vi "Page_Advanced_Initialize.vi"(6 "ctl references":T1, 8 "error in (no error)":errorcluster, 11 "AB_Application in":refnum<class "AB_Application.lvclass">) -> (0 "error out":errorcluster, 3 "AB_Application out":refnum<class "AB_Application.lvclass">)   [LabVIEW 2020, in "AB_Application.lvclass"]
uses:
  <vilib>/AppBuilder/AB_Classes/Application/AB_Application.lvclass
  e:/builds/penguin/labview/branches/2020/dev/dist/vi.lib/AppBuilder/AB_Classes/Build/AB_Build.lvclass
  <resource>/Framework/Providers/Builds/AppBuilder/AB_UI_Page_Advanced_References.ctl
  <vilib>/AppBuilder/AB_Classes/Application/AB_Application.lvclass/AB_Application.ctl
  <resource>/Framework/Providers/Common/provcom_StringGlobals.vi
  <vilib>/AppBuilder/AB_Classes/TargetFile/AB_Targetfile.lvclass
  <vilib>/AppBuilder/AB_Classes/Build/AB_Build.lvclass
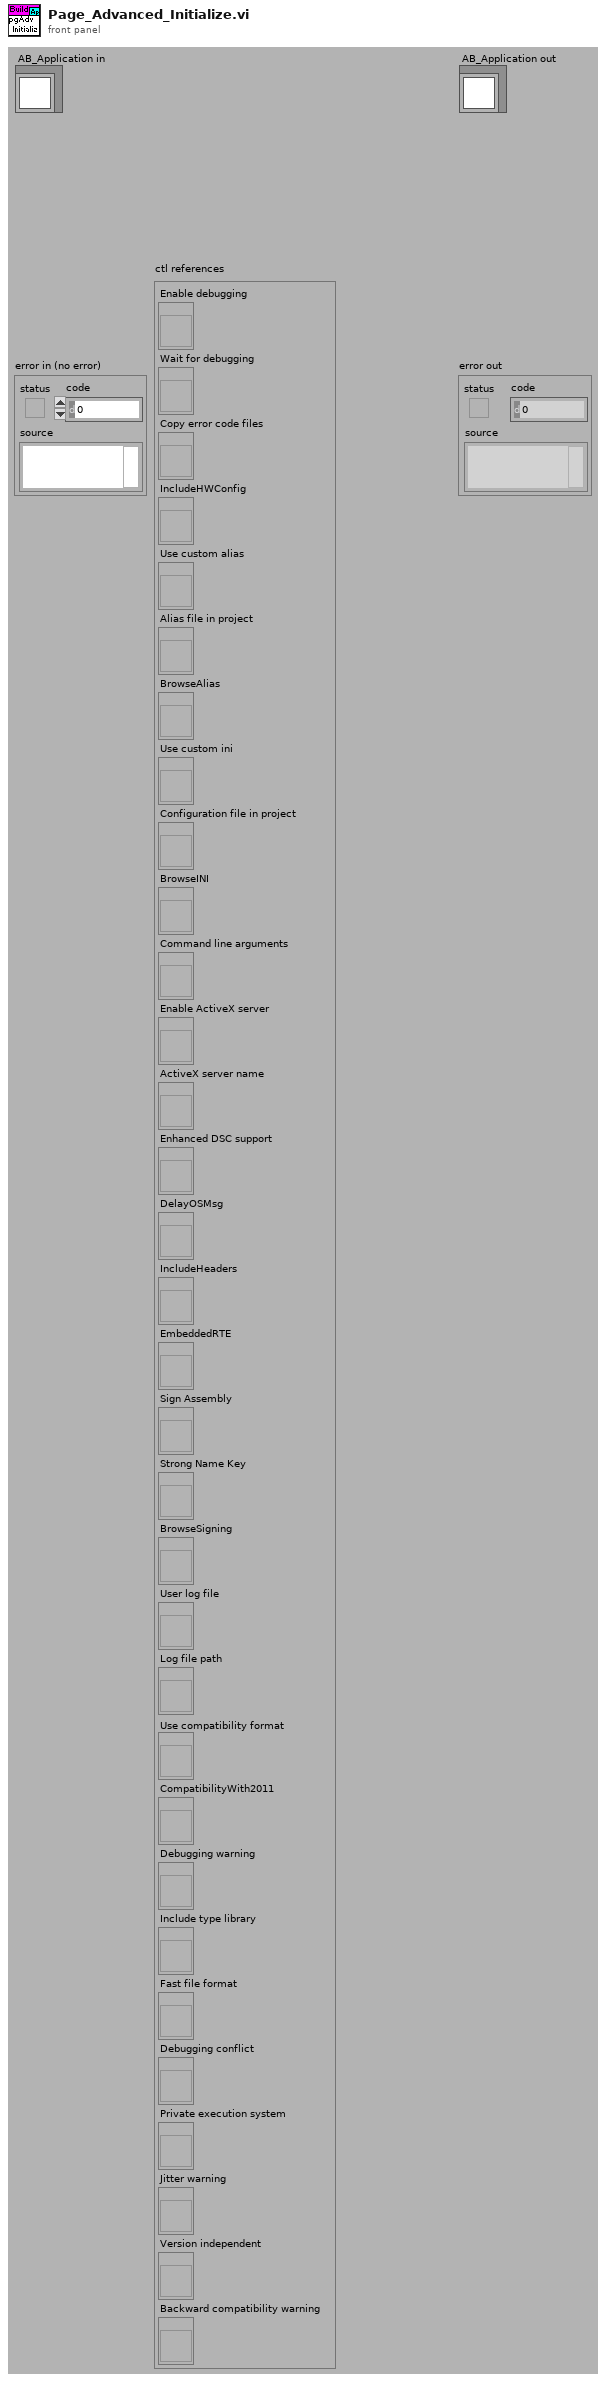
[diagram p1: front panel]
types:
  T1 = typedef "AB_UI_Page_Advanced_References.ctl" = cluster{"Enable debugging":refnum<vi>, "Wait for debugging":refnum<vi>, "Copy error code files":refnum<vi>, "IncludeHWConfig":refnum<vi>, "Use custom alias":refnum<vi>, "Alias file in project":refnum<vi>, "BrowseAlias":refnum<vi>, "Use custom ini":refnum<vi>, "Configuration file in project":refnum<vi>, "BrowseINI":refnum<vi>, "Command line arguments":refnum<vi>, "Enable ActiveX server":refnum<vi>, "ActiveX server name":refnum<vi>, "Enhanced DSC support":refnum<vi>, "DelayOSMsg":refnum<vi>, "IncludeHeaders":refnum<vi>, "EmbeddedRTE":refnum<vi>, "Sign Assembly":refnum<vi>, "Strong Name Key":refnum<vi>, "BrowseSigning":refnum<vi>, "User log file":refnum<vi>, "Log file path":refnum<vi>, "Use compatibility format":refnum<vi>, "CompatibilityWith2011":refnum<vi>, "Debugging warning":refnum<vi>, "Include type library":refnum<vi>, "Fast file format":refnum<vi>, "Debugging conflict":refnum<vi>, "Private execution system":refnum<vi>, "Jitter warning":refnum<vi>, "Version independent":refnum<vi>, "Backward compatibility warning":refnum<vi>}
  T2 = enum32{"invalid OS target", "Mac OS", "Windows 3.1", "Windows 95/NT", "Solaris 1", "Solaris 2", "HP-UX", "PowerMAX", "Linux", "Irix", "Rhapsody", "BeOS", "AIX", "OSF1", "VxWorks", "PharLap", "Carbon", "RTX", "Windows x64", "Linux x64", "Mac OS X x64"}
  T3 = typedef "AB_Build.ctl" = cluster{"buildSpecName":string, "buildSpecDescription":string, "destinations":refnum<class "AB_Destination.lvclass">[], "exclusionOption":T4, "defaultLanguage":string, "supportedLanguages":string[], "excludedDirectories":path[], "buildContext":refnum<vi>, "buildObject":T5, "preview":bool, "programatic":bool, "progressBarEvents":T6, "userLog_Path":path, "preActionID":string, "preAction_Path":path, "postActionID":string, "postAction_Path":path, "eng_checkForBrokenVIs?":bool, "eng_verboseLinkerErrors?":bool, "localDest_Path":path, "targetDest_Path":path, "removeVIObject":u16, "cache":refnum<class "PreviewCache.lvclass">, "use cache":bool, "previewCache_ID":string, "buildCache_ID":string, "eng_TempLocalDest_Path":path, "eng_collectDependencies?":bool, "versionInfo":cluster{"buildVersion":cluster{"major":u16, "minor":u16, "patch":u16, "build":u16}, "autoIncrement":bool}, "eng_enableVIChecksums":bool}
  T4 = typedef "AB_Exclusion_Option.ctl" = cluster{"typedefs":bool, "polymorphicVIs":bool, "unusedLibraryItems":bool, "modifyLibraryFile":bool, "edit-timeDependencies":bool, "inlineVIs":bool, "dependent PPLs":bool, "dependent DLLs":bool}
  T5 = typedef "ItemRef.ctl" = u64
  T6 = typedef "provcom_ProgressBar_Events.ctl" = cluster{"newJob":refnum<user-event>, "newItem":refnum<user-event>, "errorMsg":T7, "cancel":refnum<user-event>}
  T7 = typedef "mxLvBuildError.ctl" = refnum<user-event>
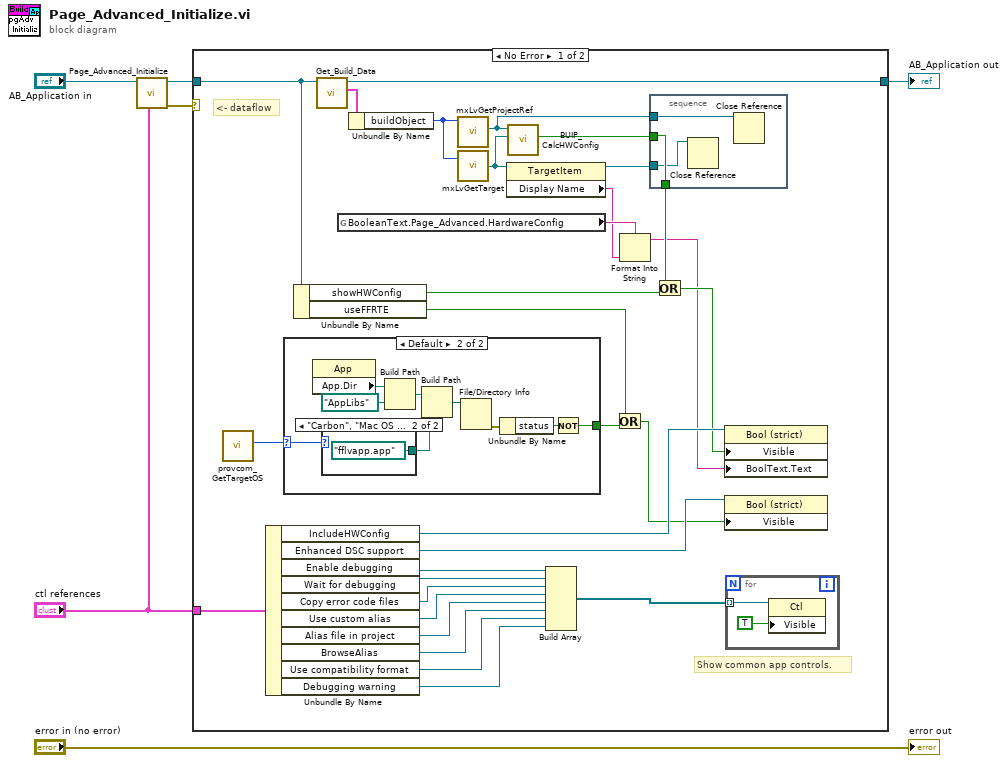
[diagram p0: block diagram]
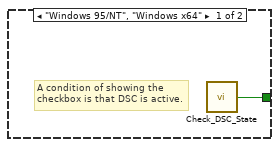
[diagram p2: hidden frame]
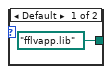
[diagram p3: hidden frame]
diagram:
  n1 = call-parent "Page_Advanced_Initialize.vi"("ctl references"="ctl references", "AB_Build in"="AB_Application in") -> ("error out"=w1:errorcluster, "AB_Build out"=w3:refnum<class "AB_Application.lvclass">)  [unwired: 1 in, 7 out]
  n2 = case shown="No Error" w1 {
    tunnel: [w34 w54] -> w5
    tunnel: w3 -> [w24 w54]
    tunnel: "ctl references" -> [w23 _]
    frame No Error {
      # "<- dataflow"
      # "Show common app controls."
      n3 = call <resource>:"provcom_GetTargetOS.vi"() -> ("App.TargetOS"=w25:T2)  [unwired: 11 out]
      n4 = Unbundle By Name(w23) -> ("IncludeHWConfig"=w32:refnum<vi>, "Enhanced DSC support"=w33:refnum<vi>, "Enable debugging"=w22:refnum<vi>, "Wait for debugging"=w21:refnum<vi>, "Copy error code files"=w20:refnum<vi>, "Use custom alias"=w19:refnum<vi>, "Alias file in project"=w18:refnum<vi>, "BrowseAlias"=w17:refnum<vi>, "Use compatibility format"=w10:refnum<vi>, "Debugging warning"=w9:refnum<vi>)
      n5 = case shown="Default" w25 {
        selector: w25 -> [_ w40]
        tunnel: [w39 w41] -> w31
        frame "Windows 95/NT", "Windows x64" {
          # "A condition of showing the checkbox is that DSC is active."
          n6 = call <vilib>:"Check_DSC_State.vi"() -> ("active"=w39:bool)  [unwired: 1 out]
        }
        frame Default {
          n7 = property class="App"() -> ("App.Dir"=w44:path)  [unwired: 2 in, 2 out]
          n8 = case shown="\"Carbon\", \"Mac OS X x64\"" w40 {
            tunnel: [path "fflvapp.lib" path "fflvapp.app"] -> w42
            frame Default {
            }
            frame "Carbon", "Mac OS X x64" {
            }
          }
          n9 = Build Path(base path=w44, name or relative path=path "AppLibs") -> (appended path=w45:path)
          n10 = Build Path(base path=w45, name or relative path=w42) -> (appended path=w46:path)
          n11 = File/Directory Info(path=w46) -> (error out=w47:errorcluster)  [unwired: 1 in, 6 out]
          n12 = Unbundle By Name(w47) -> ("status"=w48:bool)
          n13 = Not(x=w48) -> (.not. x?=w41:bool)
        }
      }
      n14 = Unbundle By Name(w24) -> ("showHWConfig"=w8:bool, "useFFRTE"=w7:bool)
      n15 = call <vilib>:"Get_Build_Data.vi"("Class in"=w24) -> ("data"=w36:T3, "Class out"=w34:refnum<class "AB_Application.lvclass">)  [unwired: 1 in, 8 out]
      n16 = global read "provcom_StringGlobals.vi" "BooleanText.Page_Advanced.HardwareConfig"() -> (w13:string)
      n17 = Unbundle By Name(w36) -> ("buildObject"=w35:T5)
      n18 = call <resource>:"mxLvGetProjectRef.vi"("Item"=w35) -> ("Project Refnum"=w26:refnum<vi>)  [unwired: 1 in, 9 out]
      n19 = call <resource>:"mxLvGetTarget.vi"("Item"=w35) -> ("Target"=w15:refnum<vi>)  [unwired: 1 in, 2 out]
      n20 = property class="TargetItem"(reference=w15) -> (reference out=w14:refnum<vi>, "Display Name"=w12:string)  [unwired: 1 in, 1 out]
      n21 = call <resource>:"BUIP_CalcHWConfig.vi"("Target"=w15, "Project"=w26) -> ("IncludeHWConfig"=w28:bool)  [unwired: 9 out]
      n22 = Build Array(w22, w21, w20, w19, w18, w17, w10, w9) -> (w16:refnum<vi>[])
      n23 = Or(x=w7, y=w31) -> (x .or. y?=w30:bool)
      n24 = Format Into String(format string=w13, w12) -> (resulting string=w11:string)  [unwired: 2 in, 1 out]
      n25 = stacked-sequence {
        tunnel: w28 -> [w53]
        tunnel: [w53] -> w27
        tunnel: w14 -> [w51]
        tunnel: w26 -> [w52]
        frame #0 {
          n26 = Close Reference(reference=w51) -> ()  [unwired: 1 in, 1 out]
          n27 = Close Reference(reference=w52) -> ()  [unwired: 1 in, 1 out]
        }
      }
      n28 = Or(x=w27, y=w8) -> (x .or. y?=w29:bool)
      n29 = property class="Bool (strict)"(reference=w32, "Visible"=w29, "BoolText.Text"=w11) -> ()  [unwired: 1 in, 2 out]
      n30 = property class="Bool (strict)"(reference=w33, "Visible"=w30) -> ()  [unwired: 1 in, 2 out]
      n31 = for {
        tunnel: w16 -> [w38] mode=indexing
        n32 = property class="Ctl"(reference=w38, "Visible"=TRUE) -> ()  [unwired: 1 in, 2 out]
      }
    }
    frame Error {
    }
  }
  "AB_Application out" <- w5
  "error out" <- "error in (no error)"
